vi "3-6.vi"() -> ()   [LabVIEW 2016]
uses:
  <vilib>/picture/picture.llb/imagedata.ctl
  <vilib>/Utility/miscctls.llb/LVBoundsTypeDef.ctl
  <vilib>/imath/engines/lvmath2/RunTimeEngine/BuiltInFunctions/zeros/NIMS_V=zeros(I32,I32).vi
  <vilib>/imath/engines/lvmath2/RunTimeEngine/ArithmeticOperatorToken/NIMS_ArithmeticOperator_power(S).vi
  <instcachedir>/0/NIMS_ArithmeticOperator_power(S)_1E6AB98FD36540B9B758A69A385A1B47.lvgen/NIMS_ArithmeticOperator_power(S)_1E6AB98FD36540B9B758A69A385A1B47_014.vi
  <vilib>/imath/engines/lvmath2/RunTimeEngine/ErrorHandling/NIMS_Create Error From Enums.vi
  <vilib>/imath/engines/lvmath2/RunTimeEngine/NodeEndStatement/NIMS_NodeEndStatement_Output.vi
  <instcachedir>/0/NIMS_NodeEndStatement_Output_53EC0D466D134D7ABD903AC30B43404B.lvgen/NIMS_NodeEndStatement_Output_53EC0D466D134D7ABD903AC30B43404B_005.vi
  <instcachedir>/0/NIMS_NodeEndStatement_Output_53EC0D466D134D7ABD903AC30B43404B.lvgen/NIMS_NodeEndStatement_Output_53EC0D466D134D7ABD903AC30B43404B_000.vi
  <vilib>/imath/engines/lvmath2/RunTimeEngine/ErrorHandling/NIMS_Finalize Error.vi
  Plot Pole-Zero - direct.vi
  Plot Frequency Response - direct.vi
  <vilib>/Analysis/3filter.llb/IIR Filter (DBL).vi
  <vilib>/Analysis/NI_AALBase.lvlib
panel:
  in  "output":path
  in  "D":dbl
  in  "use dB":bool
  out "Magnitude":cluster{dbl[], dbl[]}(graph)
  out "Pole-Zero Plot":cluster{dbl[], dbl[]}[](graph)
  in  "R":dbl
  in  "DC":dbl
  in  "write":bool
  out "new picture":picture
  out "Old Picture":picture
  out "image data":T1
  in  "input":path
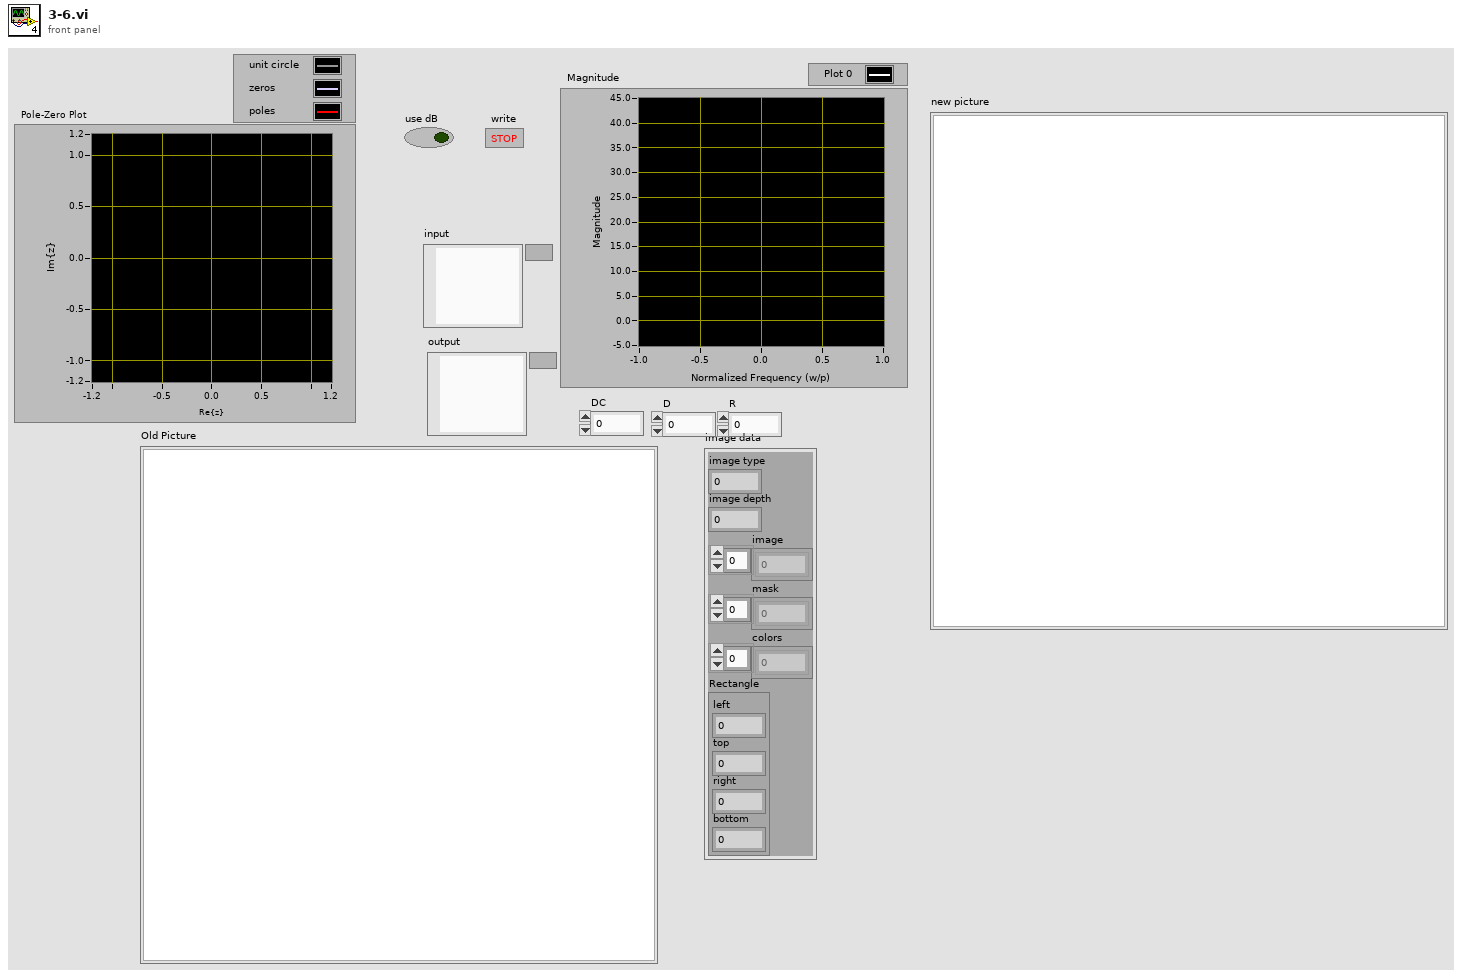
[diagram p1: front panel]
types:
  T1 = typedef "imagedata.ctl" = cluster{"image type":i32, "image depth":i32, "image":u8[], "mask":u8[], "colors":u32[], "Rectangle":cluster{"left":i16, "top":i16, "right":i16, "bottom":i16}}
  T2 = typedef "LVBoundsTypeDef.ctl" = cluster{"Width":u32, "Height":u32}
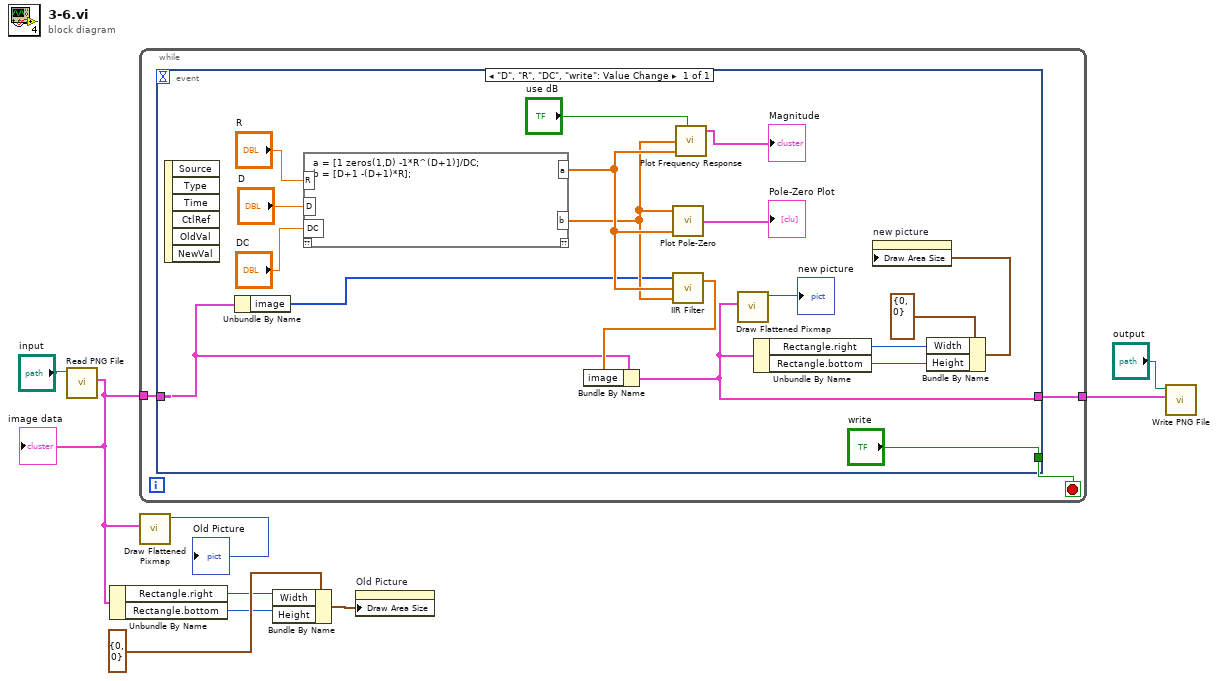
[diagram p0: block diagram]
diagram:
  n1 = call <vilib>:"Read PNG File.vi"("path to PNG file"="input") -> ("image data"=w3:T1)  [unwired: 8 in, 2 out]
  "image data" <- w3
  n2 = Unbundle By Name(w3) -> ("Rectangle.right"=w5:i16, "Rectangle.bottom"=w4:i16)
  n3 = while {
    tunnel: w3 -> [w12]
    tunnel: [w10] -> w2
    stop <- w11 stop-if-true
    n4 = event shown="[0] \"D\", \"R\", \"DC\", \"write\": Value Change" {
      selector: _ -> [_]
      dyn-events: _ -> [_]
      timeout: _ -> [_]
      tunnel: w12 -> [w22]
      tunnel: ["write"] -> w11
      tunnel: [w17] -> w10
      event "D", "R", "DC", "write": Value Change {
        n5 = event-data() -> ()  [unwired: 1 in, 6 out]
        n6 = Unbundle By Name(w22) -> ("image"=w24:u8[])
        n7 = mathscript code="a = [1 zeros(1,D) -1*R^(D+1)]/DC;\nb = [D+1 -(D+1)*R];"("D"="D", "R"="R", "DC"="DC") -> ("a"=w28:cdb[], "b"=w27:dbl[])  [unwired: 1 in, 1 out]
        n8 = call-poly "Plot Pole-Zero.vi"("a, reverse coefficients"=w28, "b, forward coefficients"=w27) -> ("Pole-Zero Plot"=→"Pole-Zero Plot":cluster{dbl[], dbl[]}[])  [unwired: 3 in]
        n9 = call-poly <vilib>:"IIR Filter.vi"("Forward Coefficients"=w27, "Reverse Coefficients"=w28, "X"=w24) -> ("Filtered X"=w23:dbl[])  [unwired: 1 in, 1 out]
        n10 = Bundle By Name(cluster=w22, "image"=w23) -> (w17:T1)
        n11 = call-poly "Plot Frequency Response.vi"("use dB"="use dB", "b, forward coefficients"=w27, "a, reverse coefficients"=w28) -> ("Magnitude"=→"Magnitude":cluster{dbl[], dbl[]})  [unwired: 2 in, 2 out]
        n12 = call <vilib>:"Draw Flattened Pixmap.vi"("image data"=w17) -> ("new picture"=→"new picture":picture)  [unwired: 8 in]
        n13 = Unbundle By Name(w17) -> ("Rectangle.right"=w19:i16, "Rectangle.bottom"=w18:i16)
        n14 = Bundle By Name(cluster=T2 {"Width"=0, "Height"=0} ("Draw Area Size"), "Width"=w19, "Height"=w18) -> (w15:T2)
        n15 = property on="new picture" class="Pict"("Draw Area Size"=w15) -> ()  [unwired: 2 in, 2 out]
      }
    }
  }
  n16 = call <vilib>:"Draw Flattened Pixmap.vi"("image data"=w3) -> ("new picture"=→"Old Picture":picture)  [unwired: 8 in]
  n17 = Bundle By Name(cluster=T2 {"Width"=0, "Height"=0} ("Draw Area Size"), "Width"=w5, "Height"=w4) -> (w6:T2)
  n18 = property on="Old Picture" class="Pict"("Draw Area Size"=w6) -> ()  [unwired: 2 in, 2 out]
  n19 = call <vilib>:"Write PNG File.vi"("image data"=w2, "path to PNG file"="output") -> ()  [unwired: 8 in, 2 out]
